vi "get_config_cluster.vi"(8 "error in (no error)":errorcluster, 11 "LightSourceMH110124MaiTai in":refnum<class "LightSourceMH110124MaiTai.lvclass">) -> (0 "error out":errorcluster, 2 "config cluster (variant)":variant, 3 "LightSourceMH110124MaiTai out":refnum<class "LightSourceMH110124MaiTai.lvclass">)   [LabVIEW 2010, in "LightSourceMH110124MaiTai.lvclass"]
uses:
  LightSourceMH110124MaiTai.lvclass
  LightSourceMH110124MaiTai.lvclass/LightSourceMH110124MaiTai.ctl
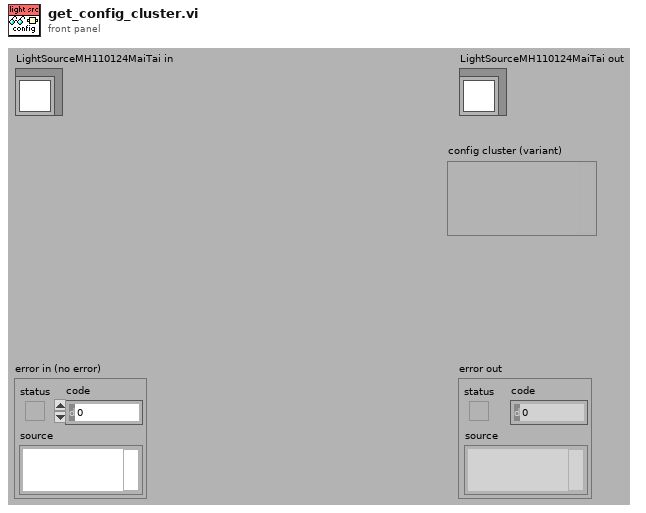
[diagram p1: front panel]
types:
  T1 = typedef "LightSourceMH110124MaiTai.lvclass/config_data_cluster.ctl" = cluster{"hardware settings":cluster{"comm port":string, "switch laser on?":bool, "open shutter?":bool, "wavelength":dbl[unit], "delay before read (ms)":u32, "flow control":u16, "stop bits":u16, "data bits":u16, "baud rate":u32, "parity (0:none)":enum16{"None", "Odd", "Even", "Mark", "Space"}}}
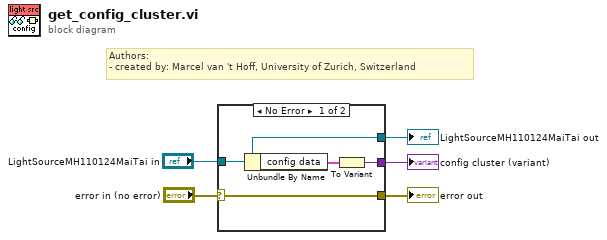
[diagram p0: block diagram]
diagram:
  # "Authors: \n- created by: Marcel van 't Hoff, University of Zurich, Switzerland"
  n1 = case shown="No Error" "error in (no error)" {
    selector: "error in (no error)" -> [w6 w10]
    tunnel: "LightSourceMH110124MaiTai in" -> [w8 w11]
    tunnel: [w8 w11] -> w2
    tunnel: [w7 _] -> w1
    tunnel: [w6 w10] -> w3
    frame No Error {
      n2 = Unbundle By Name(w8) -> ("config data"=w9:T1)
      n3 = To Variant(anything=w9) -> (Variant=w7:variant)
    }
    frame Error {
    }
  }
  "error out" <- w3
  "LightSourceMH110124MaiTai out" <- w2
  "config cluster (variant)" <- w1
